vi "Prepare miscData.vi"(8 "checksums":string[](array[string]), 9 "new":path[](array[path]), 10 "original":path[](array[path]), 11 "data in":variant) -> (3 "data out":variant)   [LabVIEW 2020, in "AB_Build.lvclass"]
uses:
  <vilib>/AppBuilder/AB_Classes/Build/AB_Build.lvclass
  <vilib>/Utility/LVLibp/NI_PackedLibraryUtility.lvlib
  <vilib>/Utility/lvfile.llb/NI_FileType.lvlib
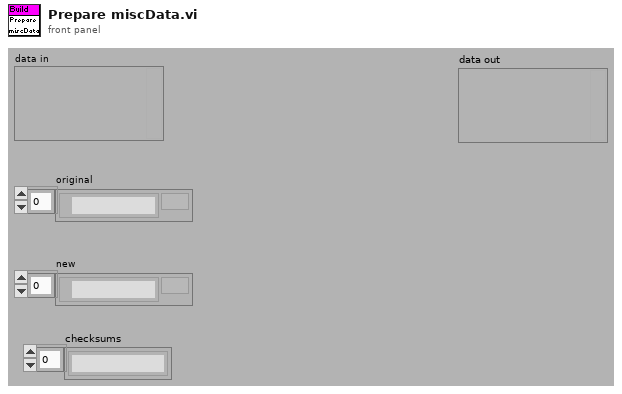
[diagram p1: front panel]
types:
  T1 = typedef "NI_FileType.lvlib/FT_FileTypes.ctl" = enum32{"Invalid file/path", "Unknown type", "Instrument", "Control", "Polymorphic VI", "Project", "Library", "LVClass", "XControl", "XNode", "CIN", "Run-time menu", "Palette menu", "LLB", "Shortcut", "Directory", "Class Private Data Control", "Statechart", "MathScript .m file", "Ladder Diagram", "LVLibp"}
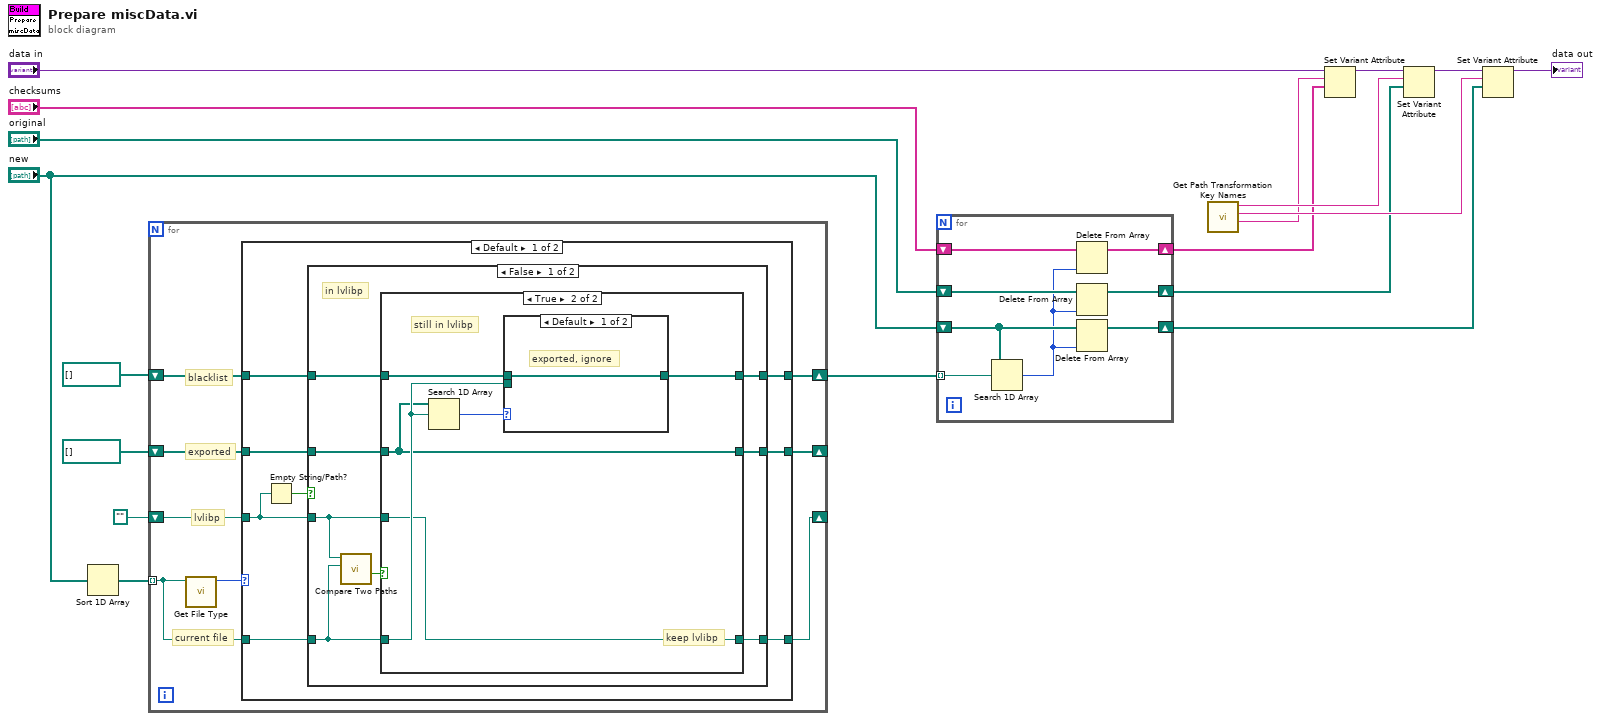
[diagram p0: block diagram]
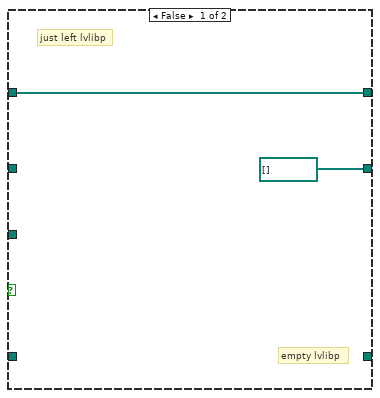
[diagram p2: hidden frame]
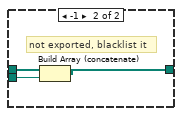
[diagram p3: hidden frame]
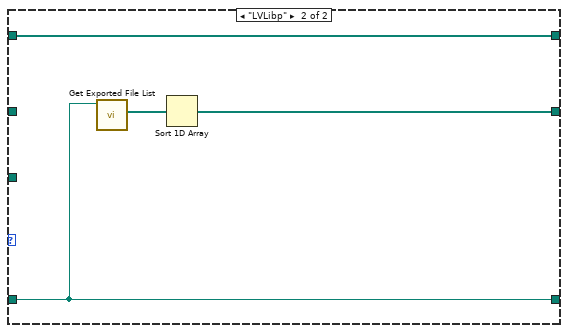
[diagram p5: hidden frame]
diagram:
  n1 = Sort 1D Array(array="new") -> (sorted array=w10:path[])
  n2 = for {
    tunnel: w10 -> [w25] mode=indexing
    shift-right: [w24] -> _
    shift-left: path "" -> [w23]
    shift-right: [w21] -> _
    shift-left: path[] [] ("new") -> [w22]
    shift-right: [w19] -> w6
    shift-left: path[] [] ("new") -> [w20]
    # "blacklist"
    # "current file"
    # "lvlibp"
    # "exported"
    n3 = call <vilib>:"Get File Type.vi"("path"=w25) -> ("file type"=w26:T1)  [unwired: 8 in, 2 out]
    n4 = case shown="Default" w26 {
      tunnel: [w30 w60] -> w24
      tunnel: w25 -> [w31 w60]
      tunnel: w23 -> [w29 _]
      tunnel: w22 -> [w33 _]
      tunnel: [w32 w58] -> w21
      tunnel: w20 -> [w28 w57]
      tunnel: [w27 w57] -> w19
      frame Default {
        n5 = Empty String/Path?(string/path=w29) -> (empty?=w34:bool)
        n6 = case shown="False" w34 {
          tunnel: [w39 w56] -> w32
          tunnel: w33 -> [w41 w56]
          tunnel: [w38 _] -> w30
          tunnel: w31 -> [w40 _]
          tunnel: w29 -> [w35 _]
          tunnel: w28 -> [w37 w55]
          tunnel: [w36 w55] -> w27
          frame False {
            # "in lvlibp"
            n7 = call <vilib>:"Compare Two Paths.vi"("Path 2"=w40, "Path 1"=w35) -> ("Path 2 Relative to Path 1?"=w42:bool)  [unwired: 6 in, 3 out]
            n8 = case shown="True" w42 {
              tunnel: w41 -> [_ w46]
              tunnel: w40 -> [_ w48]
              tunnel: [path[] [] ("new") w46] -> w39
              tunnel: [_ w45] -> w38
              tunnel: w37 -> [w43 w49]
              tunnel: [w43 w47] -> w36
              tunnel: w35 -> [_ w45]
              frame False {
                # "empty lvlibp"
                # "just left lvlibp"
              }
              frame True {
                # "keep lvlibp"
                # "still in lvlibp"
                n9 = Search 1D Array(1D array=w46, element=w48) -> (index of element=w50:i32)  [unwired: 1 in]
                n10 = case shown="Default" w50 {
                  tunnel: w49 -> [w51 w54]
                  tunnel: w48 -> [_ w53]
                  tunnel: [w51 w52] -> w47
                  frame Default {
                    # "exported, ignore"
                  }
                  frame -1 {
                    # "not exported, blacklist it"
                    n11 = Build Array (concatenate)(w54, w53) -> (w52:path[])
                  }
                }
              }
            }
          }
          frame True {
            # "not in lvlibp"
          }
        }
      }
      frame "LVLibp" {
        n12 = call <vilib>:"Get Exported File List.vi"("packed library path"=w60) -> ("paths"=w59:path[])  [unwired: 8 in, 2 out]
        n13 = Sort 1D Array(array=w59) -> (sorted array=w58:path[])
      }
    }
  }
  n14 = for {
    tunnel: w6 -> [w68] mode=indexing
    shift-right: [w65] -> w12
    shift-left: "new" -> [w64]
    shift-right: [w66] -> w13
    shift-left: "original" -> [w67]
    shift-right: [w62] -> w2
    shift-left: "checksums" -> [w63]
    n15 = Search 1D Array(1D array=w64, element=w68) -> (index of element=w61:i32)  [unwired: 1 in]
    n16 = Delete From Array(array=w63, index=w61) -> (array with subset deleted=w62:string[])  [unwired: 1 in, 1 out]
    n17 = Delete From Array(array=w67, index=w61) -> (array with subset deleted=w66:path[])  [unwired: 1 in, 1 out]
    n18 = Delete From Array(array=w64, index=w61) -> (array with subset deleted=w65:path[])  [unwired: 1 in, 1 out]
  }
  n19 = call <vilib>:"Get Path Transformation Key Names.vi"() -> ("VI Checksums"=w1:string, "New Paths Key"=w15:string, "Original Paths Key"=w18:string)  [unwired: 9 in]
  n20 = Set Variant Attribute(Variant="data in", name=w1, value=w2) -> (Variant out=w3:variant)  [unwired: 1 in, 2 out]
  n21 = Set Variant Attribute(Variant=w3, name=w18, value=w13) -> (Variant out=w17:variant)  [unwired: 1 in, 2 out]
  n22 = Set Variant Attribute(Variant=w17, name=w15, value=w12) -> (Variant out=→"data out":variant)  [unwired: 1 in, 2 out]
